vi "AI Status to Cluster.vi"(1 "AI Status Register":u16) -> (0 "AI Status Cluster":T1)   [LabVIEW 2024]
doc: "Convert AI status register value to boolean cluster."
uses:
  AI Status Cluster.ctl
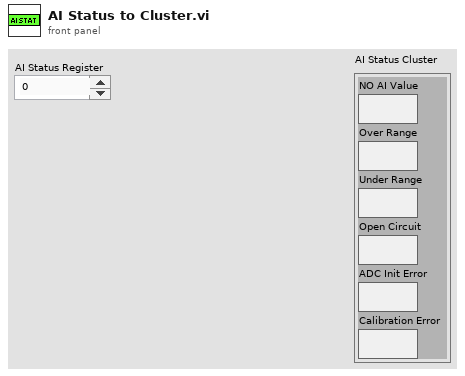
[diagram p1: front panel]
types:
  T1 = typedef "AI Status Cluster.ctl" = cluster{"NO AI Value":bool, "Over Range":bool, "Under Range":bool, "Open Circuit":bool, "ADC Init Error":bool, "Calibration Error":bool}
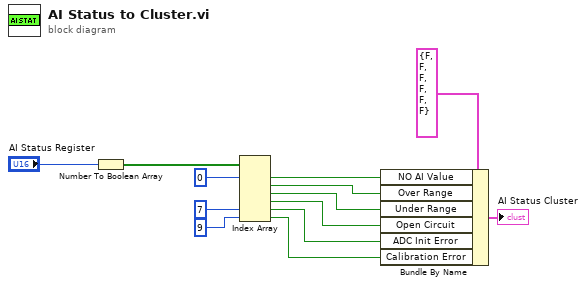
[diagram p0: block diagram]
diagram:
  n1 = Number To Boolean Array(number="AI Status Register") -> (Boolean array=w11:bool[])
  n2 = Index Array(array=w11, index #1=0 ("index"), index #5=7 ("index"), index #6=9 ("index")) -> (element #1=w9:bool, element #2=w8:bool, element #3=w7:bool, element #4=w6:bool, element #5=w4:bool, element #6=w2:bool)  [unwired: 3 in]
  n3 = Bundle By Name(cluster=T1 {"NO AI Value"=FALSE, "Over Range"=FALSE, "Under Range"=FALSE, "Open Circuit"=FALSE, "ADC Init Error"=FALSE, "Calibration Error"=FALSE} ("Cluster"), "NO AI Value"=w9, "Over Range"=w8, "Under Range"=w7, "Open Circuit"=w6, "ADC Init Error"=w4, "Calibration Error"=w2) -> (→"AI Status Cluster":T1)
